vi "ECUComms.SendandReceive.vi"(8 "error in (no error)":errorcluster, 10 "Request ID":string, 11 "Connection Ref":refnum<k5>) -> (0 "error out":errorcluster, 2 "Response":string, 3 "Connection Ref out":refnum<k5>)   [LabVIEW 2024, in "Shared Steps.lvlib"]
uses:
  Shared Steps.lvlib
  <vilib>/numeric/Random Number (Range) DBL.vi
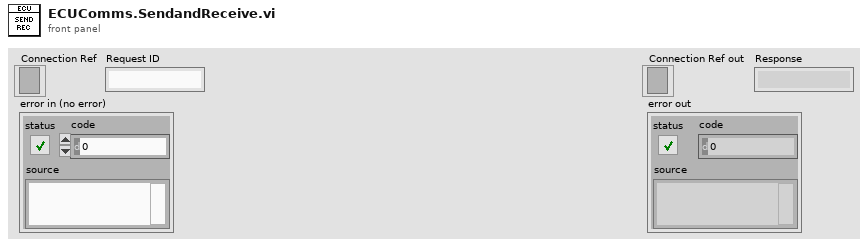
[diagram p1: front panel]
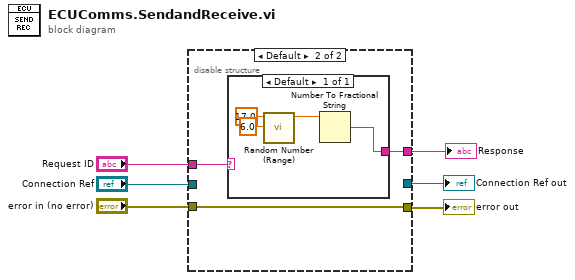
[diagram p0: block diagram]
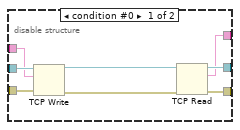
[diagram p2: hidden frame]
diagram:
  n1 = disable-structure shown="Default" {
    disable-tunnel: "Connection Ref" -> [w14 _]
    disable-tunnel: [w12 _] -> w5
    disable-tunnel: "error in (no error)" -> [w11 w15]
    disable-tunnel: [w10 w15] -> w3
    disable-tunnel: "Request ID" -> [w8 w17]
    disable-tunnel: [w7 w16] -> w1
    frame condition #0 {
      n2 = TCP Write(connection ID=w14, data in=w8, error in (no error)=w11) -> (connection ID out=w13:refnum<k5>, error out=w9:errorcluster)  [unwired: 1 in, 1 out]
      n3 = TCP Read(connection ID=w13, error in (no error)=w9) -> (connection ID out=w12:refnum<k5>, data out=w7:string, error out=w10:errorcluster)  [unwired: 3 in]
    }
    frame condition #1 (active) {
      n4 = case shown="Default" w17 {
        tunnel: [w20] -> w16
        frame Default {
          n5 = call-poly <vilib>:"Random Number (Range).vi"("lower bound (0)"=6.0, "upper bound (100)"=17.0) -> ("number"=w21:dbl)  [unwired: 9 in]
          n6 = Number To Fractional String(number=w21) -> (F-format string=w20:string)  [unwired: 3 in]
        }
      }
    }
  }
  "Connection Ref out" <- w5
  "error out" <- w3
  "Response" <- w1
